vi "Autonomous_Load.vi"(0 "Number of Commands":i32, 5 "Subsystems":string[](array[string]), 7 "Commands":string[](array[string]), 9 "Inputs":string[][](array[string]), 11 "error in":errorcluster) -> (4 "Queue_Key":refnum<queue>, 6 "Autonomous_Queue":refnum<queue>, 15 "errror out":errorcluster)   [LabVIEW 2020]
uses:
  Queue_Key_Data.ctl
  Robot_Subsystems.ctl
  Subsystems/Drive/Drive_Cluster.ctl
  Subsystems/Drive/Drive_Control_States.ctl
  Subsystems/Drive/Drive_Orientation_States.ctl
  Subsystems/Climber/Climber_Cluster.ctl
  Subsystems/Climber/Climber_Control_States.ctl
  Systems/Feeder/Feeder_Cluster.ctl
  Systems/Feeder/Feeder_Control_States.ctl
  Systems/Shooter/Determiner/Shooter_Cluster.ctl
  Systems/Shooter/Determiner/Shooter_Control_States.ctl
  a62b5066-00eb-4662-8a08-d31c7223f507.vi
  653f8947-856a-4897-9cb5-aed19e4034b9.vi
  8245bbc8-9f10-4219-b852-3f8342814532.vi
  aa76a67a-5bbd-4374-9b59-271452ffadf5.vi
  <vilib>/Comparison/Equal/Equal Functor/Equal Functor.lvclass
panel:
  out "Inputs 2":string[][](array[string])
  # "AUTO:"
  # "AUTO:"
  # "AUTO STUFF:"
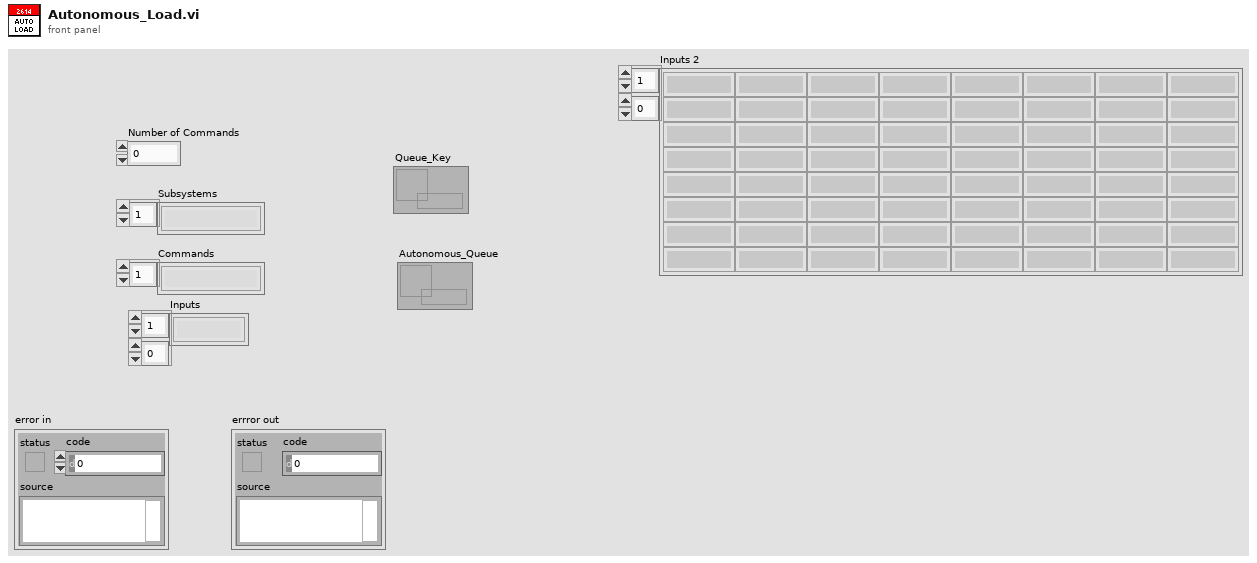
[diagram p1: front panel]
types:
  T1 = typedef "Robot_Subsystems.ctl" = cluster{"Drive_Cluster":T2, "Climber_Cluster":T5, "Feeder_Cluster":T7, "Shooter_Cluster":T9}
  T2 = typedef "Drive_Cluster.ctl" = cluster{"Control_State":T3, "Vertical_Throttle":dbl, "Lateral_Throttle":dbl, "Rotational_Throttle":dbl, "Strafe_In_Deadband":bool, "Rotation_In_Deadband":bool, "Orientation_State":T4, "Parameters":dbl[], "Step":i32, "Auto_Notifier":refnum<notifier>, "PathName":string}
  T3 = typedef "Drive_Control_States.ctl" = enum16{"No-Op", "Manual_Control", "Command_DriveDistanceAtAngle", "Command_DrivePath", "Command_SetRobotPose", "Command_Rotate", "Go_To_X"}
  T4 = typedef "Drive_Orientation_States.ctl" = enum16{"Robot-Oriented", "Field-Oriented"}
  T5 = typedef "Climber_Cluster.ctl" = cluster{"Control_State":T6, "Outer_Arm_Pivot_Throttle":dbl, "Outer_Arm_Elevator_Throttle":dbl, "Inner_Arm_Pivot_Throttle":dbl, "Enable_Climber_Sequence":bool, "Parameters":dbl[], "Auto_Notifier":refnum<notifier>, "Step":i32, "Advance_Sequencer_Step":bool}
  T6 = typedef "Climber_Control_States.ctl" = enum16{"No-Op", "Manual_%Vbus", "Correct_Outer_Pivot_Offset", "Climbing_Sequence", "Tune_PIDs", "Command_MoveArmsToSafety"}
  T7 = typedef "Feeder_Cluster.ctl" = cluster{"Firing":bool, "Load":bool, "Magazine_%Vbus":dbl, "Funnel_%Vbus":dbl, "Intake_%Vbus":dbl, "Manual_Extend":bool, "Outtake":bool, "Parameters":dbl[], "Auto_Notifier":refnum<notifier>, "Step":i32, "Control_States":T8, "Puke?":bool}
  T8 = typedef "Feeder_Control_States.ctl" = enum16{"No-Op", "Manual", "Load", "Outtake", "Firing", "Test", "Command_Feed", "Command_Shoot", "Puke-Op"}
  T9 = typedef "Shooter_Cluster.ctl" = cluster{"Control_State":T10, "Shooting?":bool, "UpperGoal?":bool, "Limelight?":bool, "Flywheel_%Vbus":dbl, "Cowl_%Vbus":dbl, "Turret_%Vbus":dbl, "Parameters":dbl[], "Auto_Notifier":refnum<notifier>, "Step":i32, "Zero_Turret":bool, "Puke?":bool}
  T10 = typedef "Shooter_Control_States.ctl" = enum16{"No-Op", "Limelight_Shooting", "Shoot_From_Pose", "Test", "Command_Shoot", "Turret_Cowl_Zero", "Manual", "Puke-Op"}
  T11 = typedef "Queue_Key_Data.ctl" = cluster{"Operation Notifier":refnum<notifier>, "Subsystem":string, "Concurrent":bool}
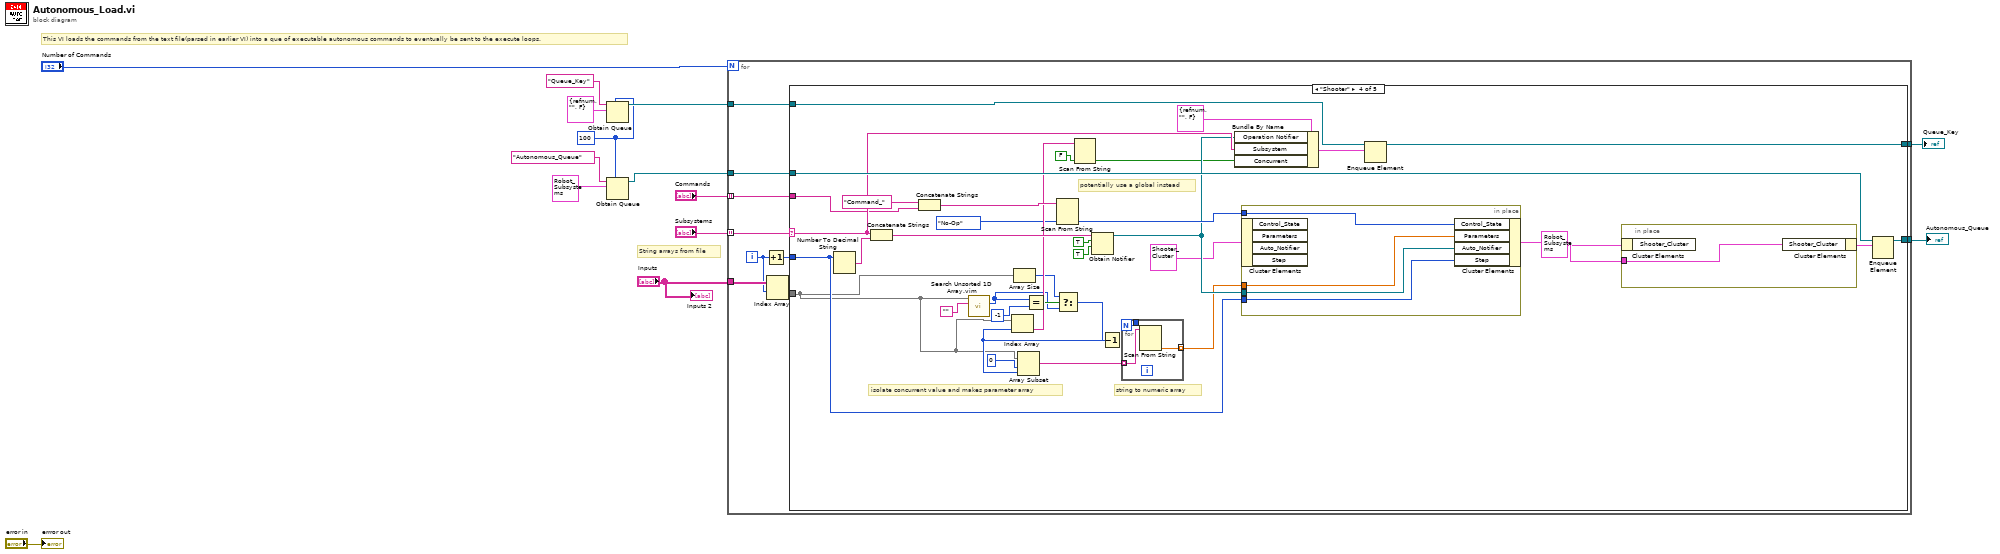
[diagram p0: block diagram]
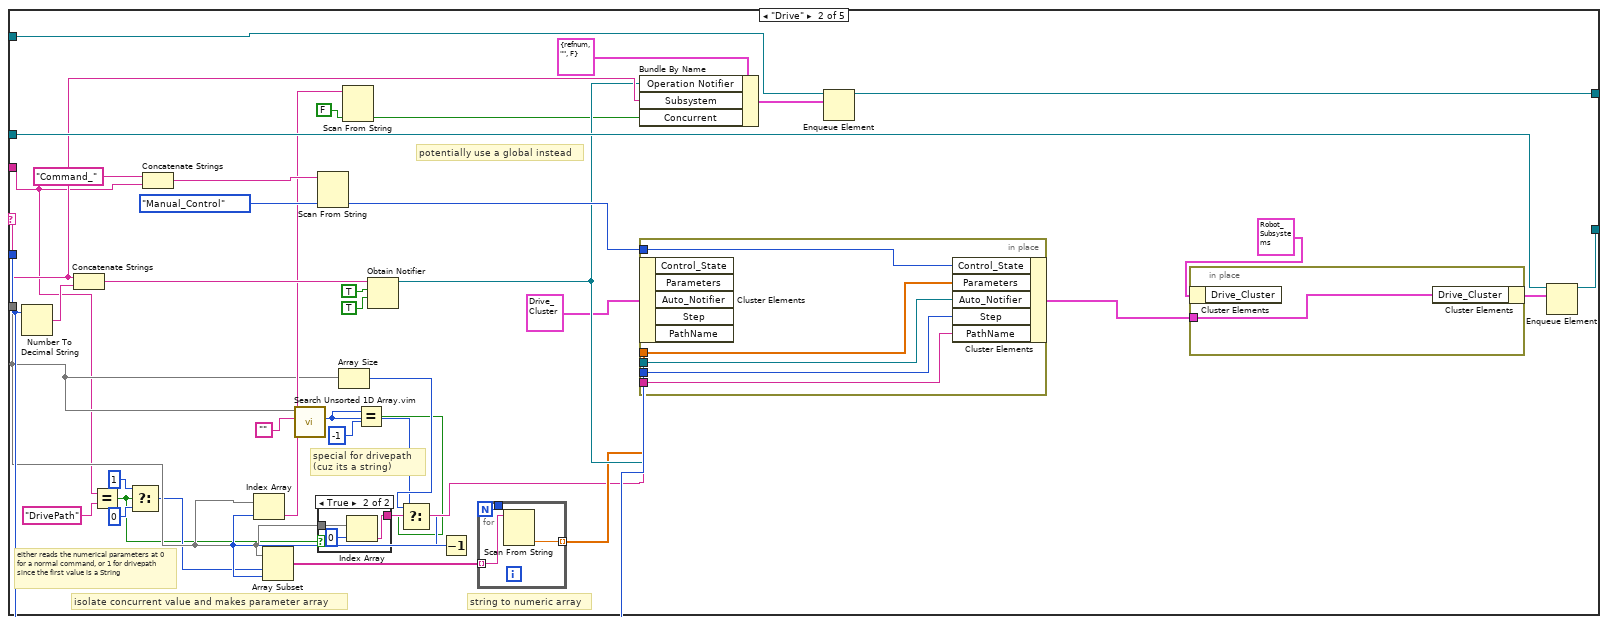
[diagram p3: hidden frame]
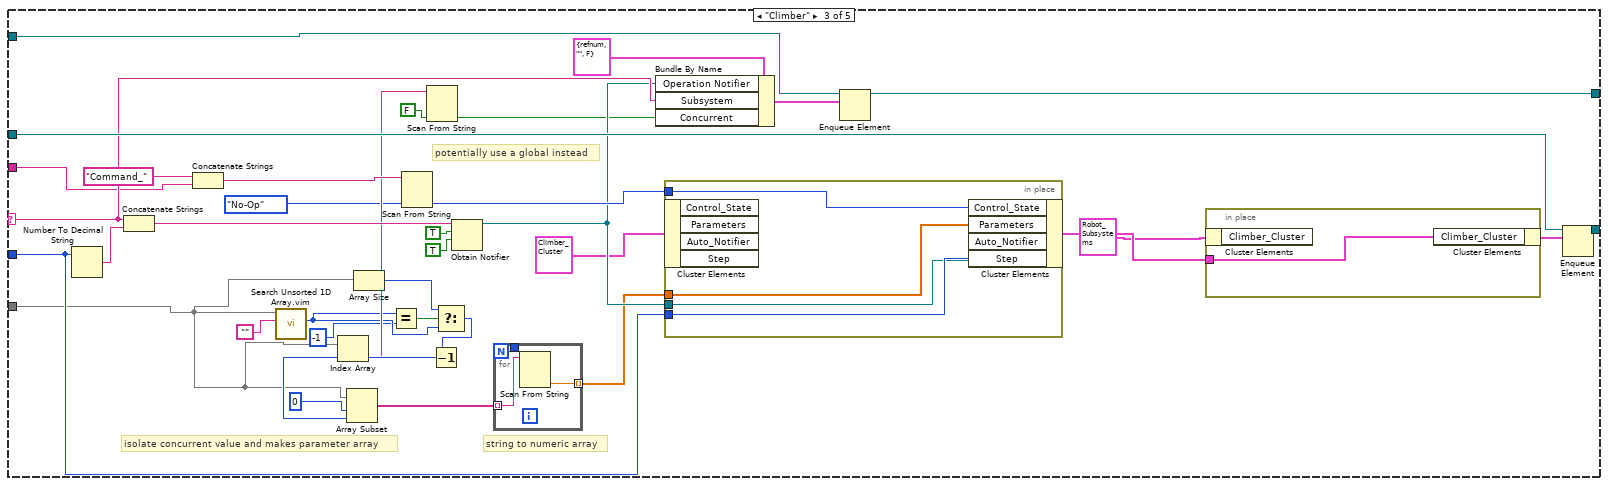
[diagram p5: hidden frame]
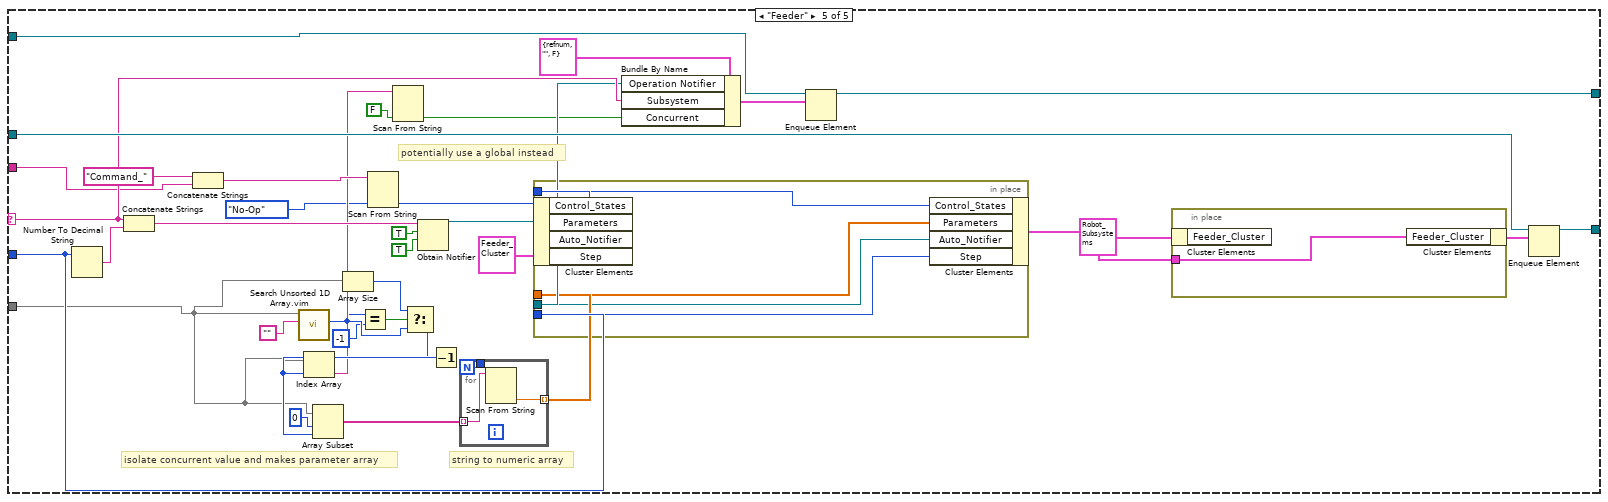
[diagram p6: hidden frame]
diagram:
  w6 = 100 ("max queue size (-1, unlimited)")
  # "This VI loads the commands from the text file(parsed in earlier VI) into a que of executable autonomous commands to eventually be sent to the execute loops."
  # "String arrays from file"
  n1 = Obtain Queue(max queue size (-1, unlimited)=w6, name (unnamed)="Queue_Key", element data type=T11 {"Operation Notifier"=refnum, "Subsystem"="", "Concurrent"=FALSE} ("Queue Key Data")) -> (queue out=w12:refnum<queue>)  [unwired: 2 in, 2 out]
  n2 = Obtain Queue(max queue size (-1, unlimited)=w6, name (unnamed)="Autonomous_Queue", element data type=T1 {"Drive_Cluster"={"Control_State"=enum."Manual_Control", "Vertical_Throttle"=0.0, "Lateral_Throttle"=0.0, "Rotational_Throttle"=0.0, "Strafe_In_Deadband"=FALSE, "Rotation_In_Deadband"=FALSE, "Orientation_State"=enum."Robot-Oriented", "Parameters"=[], "Step"=0, "Auto_Notifier"=refnum, "PathName"=""}, "Climber_Cluster"={"Control_State"=enum."No-Op", "Outer_Arm_Pivot_Throttle"=0.0, "Outer_Arm_Elevator_Throttle"=0.0, "Inner_Arm_Pivot_Throttle"=0.0, "Enable_Climber_Sequence"=FALSE, "Parameters"=[], "Auto_Notifier"=refnum, "Step"=0, "Advance_Sequencer_Step"=FALSE}, "Feeder_Cluster"={"Firing"=FALSE, "Load"=FALSE, "Magazine_%Vbus"=0.0, "Funnel_%Vbus"=0.0, "Intake_%Vbus"=0.0, "Manual_Extend"=FALSE, "Outtake"=FALSE, "Parameters"=[], "Auto_Notifier"=refnum, "Step"=0, "Control_States"=enum."No-Op", "Puke?"=FALSE}, "Shooter_Cluster"={"Control_State"=enum."No-Op", "Shooting?"=FALSE, "UpperGoal?"=FALSE, "Limelight?"=FALSE, "Flywheel_%Vbus"=0.0, "Cowl_%Vbus"=0.0, "Turret_%Vbus"=0.0, "Parameters"=[], "Auto_Notifier"=refnum, "Step"=0, "Zero_Turret"=FALSE, "Puke?"=FALSE}}) -> (queue out=w7:refnum<queue>)  [unwired: 2 in, 2 out]
  n3 = for {
    N: "Number of Commands" -> [_]
    tunnel: w12 -> [w24]
    tunnel: "Subsystems" -> [w23] mode=indexing
    tunnel: "Commands" -> [w22] mode=indexing
    tunnel: "Inputs" -> [w18]
    tunnel: [w21] -> w4
    tunnel: w7 -> [w20]
    tunnel: [w15] -> w1
    i -> [w16]
    n4 = Increment(x=w16) -> (x+1=w19:i32)
    n5 = Index Array(array=w18, index (row)=w16) -> (element=w17:string[])  [unwired: 1 in]
    n6 = case shown="\"Shooter\"" w23 {
      selector: w23 -> [_ w54 w102 w146 w190]
      tunnel: w24 -> [w25 w57 w105 w149 w193]
      tunnel: w22 -> [_ w38 w96 w140 w184]
      tunnel: [w26 w58 w106 w150 w194] -> w15
      tunnel: [w25 w50 w98 w142 w186] -> w21
      tunnel: w20 -> [w26 w61 w109 w153 w197]
      tunnel: w19 -> [_ w62 w110 w154 w198]
      tunnel: w17 -> [_ w41 w89 w133 w177]
      frame "No Op", Default {
      }
      frame "Drive" {
        # "either reads the numerical parameters at 0 for a normal command, or 1 for drivepath since the first value is a String"
        # "special for drivepath (cuz its a string)"
        # "isolate concurrent value and makes parameter array"
        # "string to numeric array"
        # "potentially use a global instead"
        n7 = Number To Decimal String(number=w62) -> (decimal integer string=w65:string)  [unwired: 1 in]
        n8 = Concatenate Strings(w54, w65) -> (w64:string)
        n9 = Equal?(x=w38, y="DrivePath") -> (x = y?=w34:bool)
        n10 = Select(t=1 ("index"), s=w34, f=0 ("index")) -> (s? t:f=w35:i32)
        n11 = Concatenate Strings("Command_" ("string"), w38) -> (w49:string)
        n12 = call "Search Unsorted 1D Array.vim"("element"="", "unsorted 1D array"=w41) -> ("index of element"=w30:i32)  [unwired: 9 in]
        n13 = Scan From String(input string=w49, default 1=Drive_Control_States."Manual_Control" ("Control_State")) -> (output 1=w63:T3)  [unwired: 3 in, 3 out]
        n14 = case shown="True" w34 {
          tunnel: w41 -> [_ w70]
          tunnel: [_ w68] -> w40
          frame False {
          }
          frame True {
            n15 = Index Array(array=w70, index=0) -> (element=w68:string)
          }
        }
        n16 = Array Size(array=w41) -> (size(s)=w32:i32)
        n17 = Equal?(x=w30, y=-1) -> (x = y?=w31:bool)
        n18 = Obtain Notifier(name (unnamed)=w64, notification data type=TRUE ("create if not found? (T)"), create if not found? (T)=TRUE) -> (notifier out=w53:refnum<notifier>)  [unwired: 1 in, 2 out]
        n19 = Select(t=w32, s=w31, f=w30) -> (s? t:f=w33:i32)
        n20 = Decrement(x=w33) -> (x-1=w45:i32)
        n21 = Index Array(array=w41, index=w45) -> (element=w44:string)
        n22 = Array Subset(array=w41, index=w35, length=w45) -> (w43:string[])
        n23 = Scan From String(input string=w44, default 1=FALSE) -> (output 1=w51:bool)  [unwired: 3 in, 3 out]
        n24 = for {
          N -> [w71]
          tunnel: w43 -> [w73] mode=indexing
          tunnel: [w72] -> w42 mode=indexing
          tunnel: [w71] -> _
          n25 = Scan From String(input string=w73) -> (output 1=w72:dbl)  [unwired: 4 in, 3 out]
        }
        n26 = Bundle By Name(cluster=T11 {"Operation Notifier"=refnum, "Subsystem"="", "Concurrent"=FALSE} ("Queue Key Data"), "Operation Notifier"=w53, "Subsystem"=w54, "Concurrent"=w51) -> (w56:T11)
        n27 = in-place {
          in-place-border: w63 -> [w77]
          in-place-border: w53 -> [w76]
          in-place-border: w62 -> [w79]
          in-place-border: w42 -> [w78]
          in-place-border: w40 -> [w75]
          n28 = in-place-cluster #1(T2 {"Control_State"=enum."Manual_Control", "Vertical_Throttle"=0.0, "Lateral_Throttle"=0.0, "Rotational_Throttle"=0.0, "Strafe_In_Deadband"=FALSE, "Rotation_In_Deadband"=FALSE, "Orientation_State"=enum."Robot-Oriented", "Parameters"=[], "Step"=0, "Auto_Notifier"=refnum, "PathName"=""} ("Drive_Cluster")) -> ()  [unwired: 5 out]
          n29 = in-place-cluster #1("Control_State"=w77, "Parameters"=w78, "Auto_Notifier"=w76, "Step"=w79, "PathName"=w75) -> (w60:T2)
        }
        n30 = Enqueue Element(queue=w57, element=w56) -> (queue out=w50:refnum<queue>)  [unwired: 2 in, 2 out]
        n31 = in-place {
          in-place-border: w60 -> [w74]
          n32 = in-place-cluster #2(T1 {"Drive_Cluster"={"Control_State"=enum."Manual_Control", "Vertical_Throttle"=0.0, "Lateral_Throttle"=0.0, "Rotational_Throttle"=0.0, "Strafe_In_Deadband"=FALSE, "Rotation_In_Deadband"=FALSE, "Orientation_State"=enum."Robot-Oriented", "Parameters"=[], "Step"=0, "Auto_Notifier"=refnum, "PathName"=""}, "Climber_Cluster"={"Control_State"=enum."No-Op", "Outer_Arm_Pivot_Throttle"=0.0, "Outer_Arm_Elevator_Throttle"=0.0, "Inner_Arm_Pivot_Throttle"=0.0, "Enable_Climber_Sequence"=FALSE, "Parameters"=[], "Auto_Notifier"=refnum, "Step"=0, "Advance_Sequencer_Step"=FALSE}, "Feeder_Cluster"={"Firing"=FALSE, "Load"=FALSE, "Magazine_%Vbus"=0.0, "Funnel_%Vbus"=0.0, "Intake_%Vbus"=0.0, "Manual_Extend"=FALSE, "Outtake"=FALSE, "Parameters"=[], "Auto_Notifier"=refnum, "Step"=0, "Control_States"=enum."No-Op", "Puke?"=FALSE}, "Shooter_Cluster"={"Control_State"=enum."No-Op", "Shooting?"=FALSE, "UpperGoal?"=FALSE, "Limelight?"=FALSE, "Flywheel_%Vbus"=0.0, "Cowl_%Vbus"=0.0, "Turret_%Vbus"=0.0, "Parameters"=[], "Auto_Notifier"=refnum, "Step"=0, "Zero_Turret"=FALSE, "Puke?"=FALSE}}) -> ()  [unwired: 1 out]
          n33 = in-place-cluster #2("Drive_Cluster"=w74) -> (w59:T1)
        }
        n34 = Enqueue Element(queue=w61, element=w59) -> (queue out=w58:refnum<queue>)  [unwired: 2 in, 2 out]
      }
      frame "Climber" {
        # "isolate concurrent value and makes parameter array"
        # "string to numeric array"
        # "potentially use a global instead"
        n35 = Number To Decimal String(number=w110) -> (decimal integer string=w113:string)  [unwired: 1 in]
        n36 = Concatenate Strings(w102, w113) -> (w112:string)
        n37 = Concatenate Strings("Command_" ("string"), w96) -> (w97:string)
        n38 = call "Search Unsorted 1D Array.vim"("element"="", "unsorted 1D array"=w89) -> ("index of element"=w83:i32)  [unwired: 9 in]
        n39 = Array Size(array=w89) -> (size(s)=w86:i32)
        n40 = Equal?(x=w83, y=-1) -> (x = y?=w84:bool)
        n41 = Scan From String(input string=w97, default 1=Climber_Control_States."No-Op" ("Control_State")) -> (output 1=w111:T6)  [unwired: 3 in, 3 out]
        n42 = Select(t=w86, s=w84, f=w83) -> (s? t:f=w85:i32)
        n43 = Decrement(x=w85) -> (x-1=w94:i32)
        n44 = Index Array(array=w89, index=w94) -> (element=w92:string)
        n45 = Array Subset(array=w89, index=0, length=w94) -> (w91:string[])
        n46 = Scan From String(input string=w92, default 1=FALSE) -> (output 1=w99:bool)  [unwired: 3 in, 3 out]
        n47 = Obtain Notifier(name (unnamed)=w112, notification data type=TRUE ("create if not found? (T)"), create if not found? (T)=TRUE) -> (notifier out=w101:refnum<notifier>)  [unwired: 1 in, 2 out]
        n48 = for {
          N -> [w116]
          tunnel: w91 -> [w118] mode=indexing
          tunnel: [w117] -> w90 mode=indexing
          tunnel: [w116] -> _
          n49 = Scan From String(input string=w118) -> (output 1=w117:dbl)  [unwired: 4 in, 3 out]
        }
        n50 = Bundle By Name(cluster=T11 {"Operation Notifier"=refnum, "Subsystem"="", "Concurrent"=FALSE} ("Queue Key Data"), "Operation Notifier"=w101, "Subsystem"=w102, "Concurrent"=w99) -> (w104:T11)
        n51 = in-place {
          in-place-border: w111 -> [w120]
          in-place-border: w101 -> [w121]
          in-place-border: w110 -> [w123]
          in-place-border: w90 -> [w122]
          n52 = in-place-cluster #3(T5 {"Control_State"=enum."No-Op", "Outer_Arm_Pivot_Throttle"=0.0, "Outer_Arm_Elevator_Throttle"=0.0, "Inner_Arm_Pivot_Throttle"=0.0, "Enable_Climber_Sequence"=FALSE, "Parameters"=[], "Auto_Notifier"=refnum, "Step"=0, "Advance_Sequencer_Step"=FALSE} ("Climber_Cluster")) -> ()  [unwired: 4 out]
          n53 = in-place-cluster #3("Control_State"=w120, "Parameters"=w122, "Auto_Notifier"=w121, "Step"=w123) -> (w108:T5)
        }
        n54 = Enqueue Element(queue=w105, element=w104) -> (queue out=w98:refnum<queue>)  [unwired: 2 in, 2 out]
        n55 = in-place {
          in-place-border: w108 -> [w119]
          n56 = in-place-cluster #4(T1 {"Drive_Cluster"={"Control_State"=enum."Manual_Control", "Vertical_Throttle"=0.0, "Lateral_Throttle"=0.0, "Rotational_Throttle"=0.0, "Strafe_In_Deadband"=FALSE, "Rotation_In_Deadband"=FALSE, "Orientation_State"=enum."Robot-Oriented", "Parameters"=[], "Step"=0, "Auto_Notifier"=refnum, "PathName"=""}, "Climber_Cluster"={"Control_State"=enum."No-Op", "Outer_Arm_Pivot_Throttle"=0.0, "Outer_Arm_Elevator_Throttle"=0.0, "Inner_Arm_Pivot_Throttle"=0.0, "Enable_Climber_Sequence"=FALSE, "Parameters"=[], "Auto_Notifier"=refnum, "Step"=0, "Advance_Sequencer_Step"=FALSE}, "Feeder_Cluster"={"Firing"=FALSE, "Load"=FALSE, "Magazine_%Vbus"=0.0, "Funnel_%Vbus"=0.0, "Intake_%Vbus"=0.0, "Manual_Extend"=FALSE, "Outtake"=FALSE, "Parameters"=[], "Auto_Notifier"=refnum, "Step"=0, "Control_States"=enum."No-Op", "Puke?"=FALSE}, "Shooter_Cluster"={"Control_State"=enum."No-Op", "Shooting?"=FALSE, "UpperGoal?"=FALSE, "Limelight?"=FALSE, "Flywheel_%Vbus"=0.0, "Cowl_%Vbus"=0.0, "Turret_%Vbus"=0.0, "Parameters"=[], "Auto_Notifier"=refnum, "Step"=0, "Zero_Turret"=FALSE, "Puke?"=FALSE}}) -> ()  [unwired: 1 out]
          n57 = in-place-cluster #4("Climber_Cluster"=w119) -> (w107:T1)
        }
        n58 = Enqueue Element(queue=w109, element=w107) -> (queue out=w106:refnum<queue>)  [unwired: 2 in, 2 out]
      }
      frame "Shooter" {
        # "isolate concurrent value and makes parameter array"
        # "string to numeric array"
        # "potentially use a global instead"
        n59 = Number To Decimal String(number=w154) -> (decimal integer string=w157:string)  [unwired: 1 in]
        n60 = Concatenate Strings(w146, w157) -> (w156:string)
        n61 = Concatenate Strings("Command_" ("string"), w140) -> (w141:string)
        n62 = call "Search Unsorted 1D Array.vim"("element"="", "unsorted 1D array"=w133) -> ("index of element"=w127:i32)  [unwired: 9 in]
        n63 = Array Size(array=w133) -> (size(s)=w129:i32)
        n64 = Equal?(x=w127, y=-1) -> (x = y?=w128:bool)
        n65 = Scan From String(input string=w141, default 1=Shooter_Control_States."No-Op" ("Shooter_Control_State")) -> (output 1=w155:T10)  [unwired: 3 in, 3 out]
        n66 = Select(t=w129, s=w128, f=w127) -> (s? t:f=w130:i32)
        n67 = Obtain Notifier(name (unnamed)=w156, notification data type=TRUE ("create if not found? (T)"), create if not found? (T)=TRUE) -> (notifier out=w145:refnum<notifier>)  [unwired: 1 in, 2 out]
        n68 = Decrement(x=w130) -> (x-1=w138:i32)
        n69 = Index Array(array=w133, index=w138) -> (element=w136:string)
        n70 = Array Subset(array=w133, index=0, length=w138) -> (w135:string[])
        n71 = Scan From String(input string=w136, default 1=FALSE) -> (output 1=w143:bool)  [unwired: 3 in, 3 out]
        n72 = for {
          N -> [w160]
          tunnel: w135 -> [w162] mode=indexing
          tunnel: [w161] -> w134 mode=indexing
          tunnel: [w160] -> _
          n73 = Scan From String(input string=w162) -> (output 1=w161:dbl)  [unwired: 4 in, 3 out]
        }
        n74 = Bundle By Name(cluster=T11 {"Operation Notifier"=refnum, "Subsystem"="", "Concurrent"=FALSE} ("Queue Key Data"), "Operation Notifier"=w145, "Subsystem"=w146, "Concurrent"=w143) -> (w148:T11)
        n75 = in-place {
          in-place-border: w155 -> [w164]
          in-place-border: w145 -> [w165]
          in-place-border: w154 -> [w167]
          in-place-border: w134 -> [w166]
          n76 = in-place-cluster #5(T9 {"Control_State"=enum."No-Op", "Shooting?"=FALSE, "UpperGoal?"=FALSE, "Limelight?"=FALSE, "Flywheel_%Vbus"=0.0, "Cowl_%Vbus"=0.0, "Turret_%Vbus"=0.0, "Parameters"=[], "Auto_Notifier"=refnum, "Step"=0, "Zero_Turret"=FALSE, "Puke?"=FALSE} ("Shooter_Cluster")) -> ()  [unwired: 4 out]
          n77 = in-place-cluster #5("Control_State"=w164, "Parameters"=w166, "Auto_Notifier"=w165, "Step"=w167) -> (w152:T9)
        }
        n78 = Enqueue Element(queue=w149, element=w148) -> (queue out=w142:refnum<queue>)  [unwired: 2 in, 2 out]
        n79 = in-place {
          in-place-border: w152 -> [w163]
          n80 = in-place-cluster #6(T1 {"Drive_Cluster"={"Control_State"=enum."Manual_Control", "Vertical_Throttle"=0.0, "Lateral_Throttle"=0.0, "Rotational_Throttle"=0.0, "Strafe_In_Deadband"=FALSE, "Rotation_In_Deadband"=FALSE, "Orientation_State"=enum."Robot-Oriented", "Parameters"=[], "Step"=0, "Auto_Notifier"=refnum, "PathName"=""}, "Climber_Cluster"={"Control_State"=enum."No-Op", "Outer_Arm_Pivot_Throttle"=0.0, "Outer_Arm_Elevator_Throttle"=0.0, "Inner_Arm_Pivot_Throttle"=0.0, "Enable_Climber_Sequence"=FALSE, "Parameters"=[], "Auto_Notifier"=refnum, "Step"=0, "Advance_Sequencer_Step"=FALSE}, "Feeder_Cluster"={"Firing"=FALSE, "Load"=FALSE, "Magazine_%Vbus"=0.0, "Funnel_%Vbus"=0.0, "Intake_%Vbus"=0.0, "Manual_Extend"=FALSE, "Outtake"=FALSE, "Parameters"=[], "Auto_Notifier"=refnum, "Step"=0, "Control_States"=enum."No-Op", "Puke?"=FALSE}, "Shooter_Cluster"={"Control_State"=enum."No-Op", "Shooting?"=FALSE, "UpperGoal?"=FALSE, "Limelight?"=FALSE, "Flywheel_%Vbus"=0.0, "Cowl_%Vbus"=0.0, "Turret_%Vbus"=0.0, "Parameters"=[], "Auto_Notifier"=refnum, "Step"=0, "Zero_Turret"=FALSE, "Puke?"=FALSE}}) -> ()  [unwired: 1 out]
          n81 = in-place-cluster #6("Shooter_Cluster"=w163) -> (w151:T1)
        }
        n82 = Enqueue Element(queue=w153, element=w151) -> (queue out=w150:refnum<queue>)  [unwired: 2 in, 2 out]
      }
      frame "Feeder" {
        # "isolate concurrent value and makes parameter array"
        # "string to numeric array"
        # "potentially use a global instead"
        n83 = Number To Decimal String(number=w198) -> (decimal integer string=w201:string)  [unwired: 1 in]
        n84 = Concatenate Strings(w190, w201) -> (w200:string)
        n85 = Concatenate Strings("Command_" ("string"), w184) -> (w185:string)
        n86 = call "Search Unsorted 1D Array.vim"("element"="", "unsorted 1D array"=w177) -> ("index of element"=w171:i32)  [unwired: 9 in]
        n87 = Array Size(array=w177) -> (size(s)=w174:i32)
        n88 = Equal?(x=w171, y=-1) -> (x = y?=w172:bool)
        n89 = Scan From String(input string=w185, default 1=Feeder_Control_States."No-Op" ("Control_States")) -> (output 1=w199:T8)  [unwired: 3 in, 3 out]
        n90 = Select(t=w174, s=w172, f=w171) -> (s? t:f=w173:i32)
        n91 = Obtain Notifier(name (unnamed)=w200, notification data type=TRUE ("create if not found? (T)"), create if not found? (T)=TRUE) -> (notifier out=w189:refnum<notifier>)  [unwired: 1 in, 2 out]
        n92 = Decrement(x=w173) -> (x-1=w182:i32)
        n93 = Index Array(array=w177, index=w182) -> (element=w180:string)
        n94 = Array Subset(array=w177, index=0, length=w182) -> (w179:string[])
        n95 = Scan From String(input string=w180, default 1=FALSE) -> (output 1=w187:bool)  [unwired: 3 in, 3 out]
        n96 = for {
          N -> [w204]
          tunnel: w179 -> [w206] mode=indexing
          tunnel: [w205] -> w178 mode=indexing
          tunnel: [w204] -> _
          n97 = Scan From String(input string=w206) -> (output 1=w205:dbl)  [unwired: 4 in, 3 out]
        }
        n98 = in-place {
          in-place-border: w199 -> [w208]
          in-place-border: w189 -> [w209]
          in-place-border: w198 -> [w211]
          in-place-border: w178 -> [w210]
          n99 = in-place-cluster #7(T7 {"Firing"=FALSE, "Load"=FALSE, "Magazine_%Vbus"=0.0, "Funnel_%Vbus"=0.0, "Intake_%Vbus"=0.0, "Manual_Extend"=FALSE, "Outtake"=FALSE, "Parameters"=[], "Auto_Notifier"=refnum, "Step"=0, "Control_States"=enum."No-Op", "Puke?"=FALSE} ("Feeder_Cluster")) -> ()  [unwired: 4 out]
          n100 = in-place-cluster #7("Control_States"=w208, "Parameters"=w210, "Auto_Notifier"=w209, "Step"=w211) -> (w196:T7)
        }
        n101 = Bundle By Name(cluster=T11 {"Operation Notifier"=refnum, "Subsystem"="", "Concurrent"=FALSE} ("Queue Key Data"), "Operation Notifier"=w189, "Subsystem"=w190, "Concurrent"=w187) -> (w192:T11)
        n102 = Enqueue Element(queue=w193, element=w192) -> (queue out=w186:refnum<queue>)  [unwired: 2 in, 2 out]
        n103 = in-place {
          in-place-border: w196 -> [w207]
          n104 = in-place-cluster #8(T1 {"Drive_Cluster"={"Control_State"=enum."Manual_Control", "Vertical_Throttle"=0.0, "Lateral_Throttle"=0.0, "Rotational_Throttle"=0.0, "Strafe_In_Deadband"=FALSE, "Rotation_In_Deadband"=FALSE, "Orientation_State"=enum."Robot-Oriented", "Parameters"=[], "Step"=0, "Auto_Notifier"=refnum, "PathName"=""}, "Climber_Cluster"={"Control_State"=enum."No-Op", "Outer_Arm_Pivot_Throttle"=0.0, "Outer_Arm_Elevator_Throttle"=0.0, "Inner_Arm_Pivot_Throttle"=0.0, "Enable_Climber_Sequence"=FALSE, "Parameters"=[], "Auto_Notifier"=refnum, "Step"=0, "Advance_Sequencer_Step"=FALSE}, "Feeder_Cluster"={"Firing"=FALSE, "Load"=FALSE, "Magazine_%Vbus"=0.0, "Funnel_%Vbus"=0.0, "Intake_%Vbus"=0.0, "Manual_Extend"=FALSE, "Outtake"=FALSE, "Parameters"=[], "Auto_Notifier"=refnum, "Step"=0, "Control_States"=enum."No-Op", "Puke?"=FALSE}, "Shooter_Cluster"={"Control_State"=enum."No-Op", "Shooting?"=FALSE, "UpperGoal?"=FALSE, "Limelight?"=FALSE, "Flywheel_%Vbus"=0.0, "Cowl_%Vbus"=0.0, "Turret_%Vbus"=0.0, "Parameters"=[], "Auto_Notifier"=refnum, "Step"=0, "Zero_Turret"=FALSE, "Puke?"=FALSE}}) -> ()  [unwired: 1 out]
          n105 = in-place-cluster #8("Feeder_Cluster"=w207) -> (w195:T1)
        }
        n106 = Enqueue Element(queue=w197, element=w195) -> (queue out=w194:refnum<queue>)  [unwired: 2 in, 2 out]
      }
    }
  }
  "Queue_Key" <- w4
  "Autonomous_Queue" <- w1
  "errror out" <- "error in"
  "Inputs 2" <- "Inputs"
